vi "Merge.vi"(0 "arr":i32, 1 "nOrder":i32, 2 "nPoint":i32, 3 "nPixel":i32, 4 "coeff":sgl, 5 "fit":i32, 6 "hbin":i32, 8 "output":i32, 9 "start":sgl, 10 "step_Renamed":sgl) -> (16 "step_Renamed out":sgl, 18 "output out":i32, 19 "start out":sgl, 20 "function return":u32, 24 "coeff out":sgl)   [LabVIEW 2018, in "Copy of Andor SDK.lvlib"]
doc: "EXPNETTYPE unsigned int WINAPI Merge(const at_32 * arr, long nOrder, long nPoint, long nPixel, float * coeff, long fit, long hbin, at_32 * output, float * start, float * step_Renamed);"
uses:
  Copy of Andor SDK.lvlib
  <userlib>/Andor SDK/ATMCD32D.dll
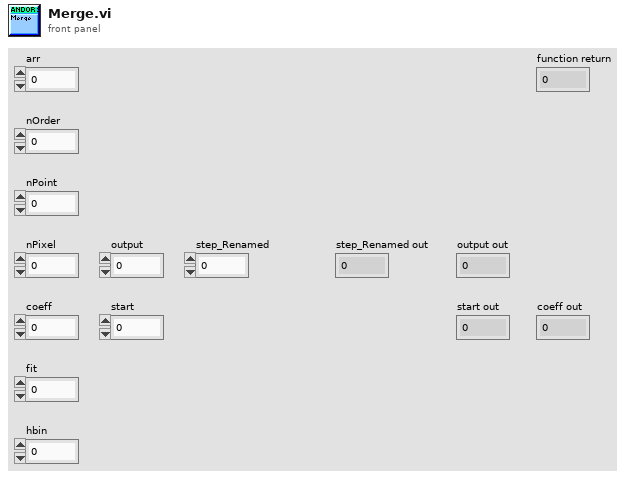
[diagram p1: front panel]
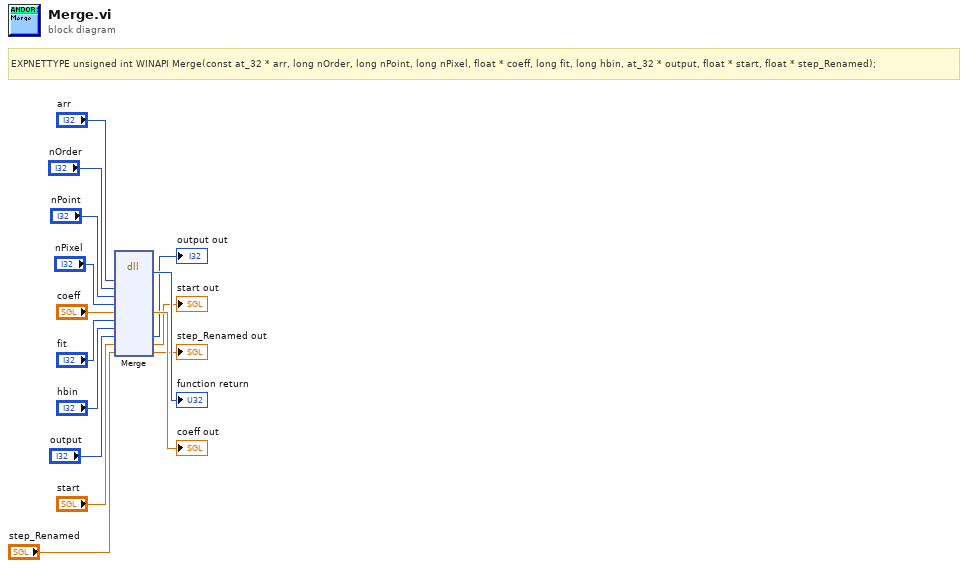
[diagram p0: block diagram]
diagram:
  # "EXPNETTYPE unsigned int WINAPI Merge(const at_32 * arr, long nOrder, long nPoint, long nPixel, float * coeff, long fit, long hbin, at_32 * output, float * start, float * step_Renamed);"
  n1 = dll-call lib="C:/Program Files (x86)/National Instruments/LabVIEW 2018/user.lib/Andor SDK/ATMCD32D.*" fn="Merge"("arr"="arr", "nOrder"="nOrder", "nPoint"="nPoint", "nPixel"="nPixel", "coeff"="coeff", "fit"="fit", "hbin"="hbin", "output"="output", "start"="start", "step_Renamed"="step_Renamed") -> (→"function return":u32, "coeff"=→"coeff out":sgl, "output"=→"output out":i32, "start"=→"start out":sgl, "step_Renamed"=→"step_Renamed out":sgl)  [unwired: 9 in, 2 out]
